vi "Show Cursors_Normal.vi"(6 "Cursor Options":T1={"font"={"Font Name"="Arial", "Size"=14, "Strikeout?"=FALSE, "Italic?"=FALSE, "Underline?"=FALSE, "Outline?"=FALSE, "Shadow?"=FALSE, "Bold?"=FALSE}, "size"=1, "Timestamp"=enum."at TOP", "Vertical Line?"=TRUE, "Horizontal Line?"=TRUE, "alignment(left, top)"={"horizontal"=enum."left", "vertical"=enum."center"}, "TextFormat"=" %3$s\\n %2$.2f", "time format (%H:%M:%S)"="%H:%M:%S"} {"size" min=1 max=50}, 7 "Index":i32, 8 "error in (no error)":errorcluster, 9 "Coords":T2, 10 "XY Graph":refnum<vi>, 11 "input picture":picture) -> (0 "error out":errorcluster, 3 "output picture":picture)   [LabVIEW 2018]
doc: "Shows real time cursors overlayed in a graph, using just one mouse move event case. The options for the cursors can be highly customized to set up a unique cursor style.\n\nUsage: Place this inside an event structure on any XY graph, in the \"Mouse Move\" event case. Set the options as an input cluster to override the defaults. The output picture control would typically be connected to the XY Graph's \"PlotImages.Front\" property item.\n\nCursor Options\n<b>Horizontal Line?</b> - Draws a horizontal line to intersect each plot\n<b>Verticle Line?</b> - Draws a verticle line at the mouse location to highlight the cursor location (typically on the time scale)\n<b>Timestamp</b> - Sets where to display the timestamp (if you want it at the top or bottom) Used best with the verticle line turned on.\n<b>Font</b> - Setup the font for displaying the cursor text\n<b>Alignment</b> - Sets the alignment options for the text relative to the cursor point\n<b>TextFormat</b> - Sets the text display format at the cursor points to show. Three input parameters are available for the text, which can be accessed using parameter numbers.\ninputs: \n1$ - Timestamp at cursor locations\n2$ - Value of the plot\n3$ - Name of the plot\n\nExamples: $2$.2f\\n\\n%1$s\nThis shows the value of the plot with 2 decimal places. A blank line, then the name of the plot"
uses:
  <vilib>/Utility/miscctls.llb/LVPoint32TypeDef.ctl
  CursorOptions.ctl
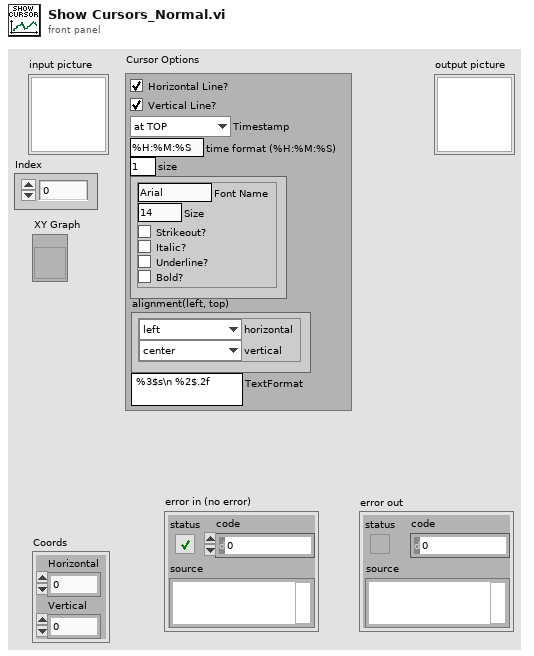
[diagram p1: front panel]
types:
  T1 = typedef "CursorOptions.ctl" = cluster{"font":cluster{"Font Name":string, "Size":i16, "Strikeout?":bool, "Italic?":bool, "Underline?":bool, "Outline?":bool, "Shadow?":bool, "Bold?":bool}, "size":i16, "Timestamp":enum16{"at TOP", "at BOTTOM", "none"}, "Vertical Line?":bool, "Horizontal Line?":bool, "alignment(left, top)":cluster{"horizontal":enum16{"left", "center", "right"}, "vertical":enum16{"top", "center", "bottom"}}, "TextFormat":string, "time format (%H:%M:%S)":string}
  T2 = typedef "LVPoint32TypeDef.ctl" = cluster{"Horizontal":i32, "Vertical":i32}
  T3 = enum16{"User-specified Font", "Application Font", "System Font", "Dialog Font"}
  T4 = cluster{"horizontal":enum16{"left", "center", "right"}, "vertical":enum16{"top", "center", "bottom"}}
  T5 = cluster{"Font Name":string, "Size":i16, "Strikeout?":bool, "Italic?":bool, "Underline?":bool, "Outline?":bool, "Shadow?":bool, "Bold?":bool}
  T6 = typedef "LVRectTypeDef.ctl" = cluster{"Left":i16, "Top":i16, "Right":i16, "Bottom":i16}
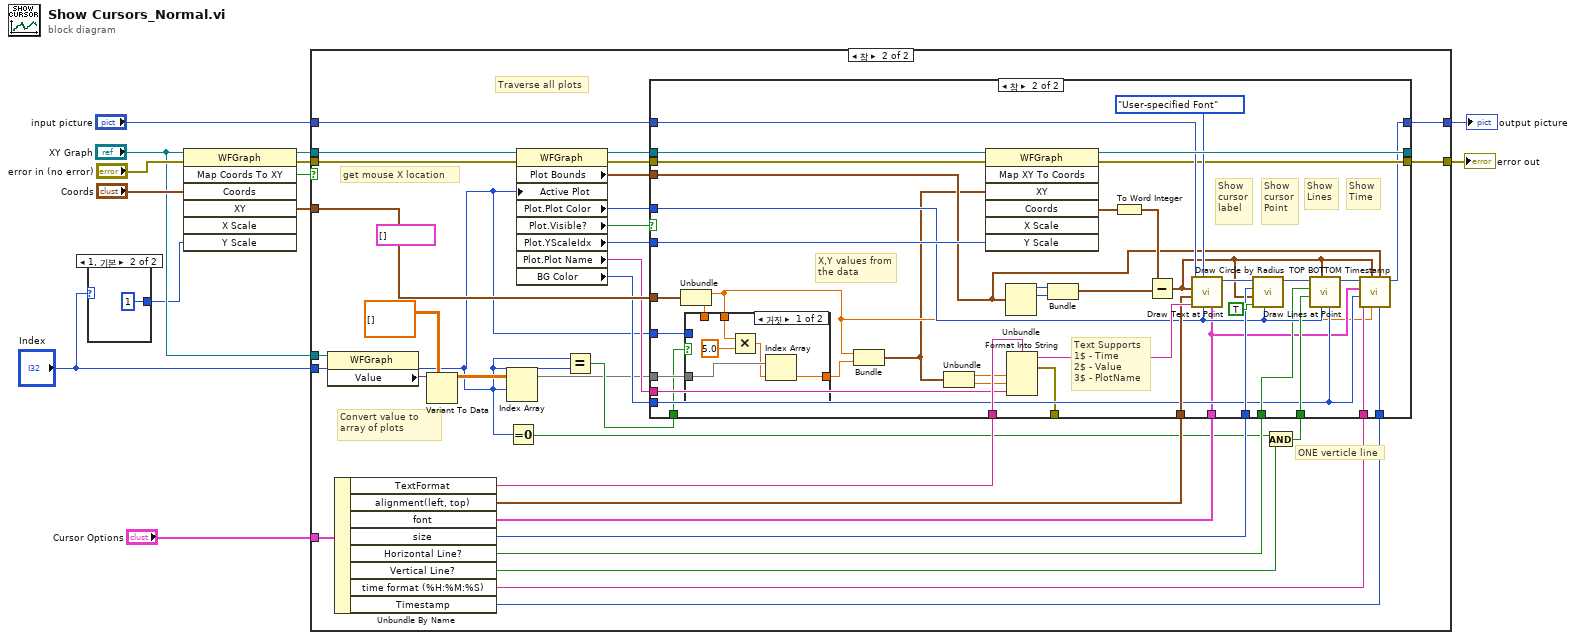
[diagram p0: block diagram]
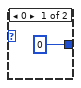
[diagram p2: hidden frame]
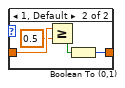
[diagram p6: hidden frame]
diagram:
  n1 = case shown="1, 기본" "Index" {
    tunnel: [0 1] -> w1
    frame 0 {
    }
    frame 1, Default {
    }
  }
  n2 = invoke on="Invoke Node" class="WFGraph" method="Map Coords To XY"(reference="XY Graph", error in="error in (no error)", "Coords"="Coords", "Y Scale"=w1) -> (reference out=w10:refnum<vi>, error out=w9:errorcluster, "Map Coords To XY"=w12:bool, "XY"=w13:cluster{"X":dbl, "Y":dbl})  [unwired: 3 in, 3 out]
  n3 = case shown="참" w12 {
    tunnel: w13 -> [_ w48]
    tunnel: w10 -> [_ w49]
    tunnel: [w16 w47] -> w5
    tunnel: w9 -> [w17 w46]
    tunnel: [w17 w45] -> w8
    tunnel: "input picture" -> [w16 w44]
    tunnel: "Cursor Options" -> [_ w36]
    tunnel: "XY Graph" -> [_ w34]
    tunnel: "Index" -> [_ w18]
    frame False {
      # "not in plot area.  clear the image"
    }
    frame True {
      (unwired) cluster{dbl[], dbl[]}[] []
      # "Traverse all plots"
      # "ONE verticle line"
      # "Convert value to array of plots"
      # "get mouse X location"
      n4 = property class="WFGraph"(reference=w34) -> ("Value"=w33:variant)  [unwired: 1 in, 2 out]
      n5 = Unbundle By Name(w36) -> ("TextFormat"=w43:string, "alignment(left, top)"=w42:T4, "font"=w41:T5, "size"=w40:i16, "Horizontal Line?"=w39:bool, "Vertical Line?"=w38:bool, "time format (%H:%M:%S)"=w32:string, "Timestamp"=w37:enum16{"at TOP", "at BOTTOM", "none"})
      n6 = Variant To Data(type=dbl[][] [], Variant=w33) -> (data=w35:dbl[][])  [unwired: 1 in, 1 out]
      n7 = Index Array(array=w35, index (row)=w18) -> (element=w19:dbl[])  [unwired: 1 in]
      n8 = Equal To 0?(x=w18) -> (x = 0?=w21:bool)
      n9 = property on="Property Node" class="WFGraph"(reference=w49, error in=w46, "Active Plot"=w18) -> (reference out=w29:refnum<vi>, error out=w26:errorcluster, "Plot Bounds"=w30:T6, "Plot.Plot Color"=w28:u32, "Plot.Visible?"=w27:bool, "Plot.YScaleIdx"=w25:u32, "Plot.Plot Name"=w23:string, "BG Color"=w22:u32)
      n10 = Equal?(x=w18, y=w18) -> (x = y?=w20:bool)
      n11 = And(x=w21, y=w38) -> (x .and. y?=w24:bool)
      n12 = case shown="참" w27 {
        tunnel: w30 -> [_ w65]
        tunnel: [w52 w89] -> _
        tunnel: w19 -> [_ w60]
        tunnel: w48 -> [_ w56]
        tunnel: w44 -> [w51 w88]
        tunnel: w29 -> [w52 w86]
        tunnel: [w51 w69] -> w47
        tunnel: w28 -> [_ w74]
        tunnel: w26 -> [w50 w82]
        tunnel: [w50 w81] -> w45
        tunnel: w25 -> [_ w80]
        tunnel: w40 -> [_ w79]
        tunnel: w42 -> [_ w78]
        tunnel: w41 -> [_ w63]
        tunnel: w43 -> [_ w77]
        tunnel: w39 -> [_ w73]
        tunnel: w24 -> [_ w76]
        tunnel: w23 -> [_ w70]
        tunnel: w37 -> [_ w67]
        tunnel: w22 -> [_ w64]
        tunnel: [_ w62] -> _
        tunnel: w32 -> [_ w61]
        tunnel: w20 -> [_ w55]
        tunnel: w18 -> [_ w53]
        frame False {
          # "plot is not visible, so don't show the cursor for it."
        }
        frame True {
          # "Show\nTime"
          # "Show\nLines"
          # "Show\ncursor\nPoint"
          # "Show\ncursor\nlabel"
          # "Text Supports\n1$ - Time\n2$ - Value\n3$ - PlotName"
          # "X,Y values from the data"
          n13 = Unbundle(w56) -> ("X"=w59:dbl, "Y"=w54:dbl)
          n14 = case shown="거짓" w55 {
            tunnel: w60 -> [w99 _]
            tunnel: w59 -> [w98 _]
            tunnel: [w95 w101] -> w58
            tunnel: w54 -> [_ w100]
            tunnel: w53 -> [_ w102]
            frame False {
              n15 = Multiply(x=w98, y=5.0) -> (x*y=w97:dbl)
              n16 = Index Array(array=w99, index=w97) -> (element=w95:dbl)
            }
            frame True {
              n17 = case shown="0" w102 {
                tunnel: [w103 w104] -> w101
                tunnel: w100 -> [w103 w107]
                frame 0 {
                }
                frame 1, Default {
                  n18 = Greater Or Equal?(x=w107, y=0.5) -> (x >= y?=w105:bool)
                  n19 = Boolean To (0,1)(Boolean=w105) -> (0, 1=w104:i16)
                }
              }
            }
          }
          n20 = Bundle("X"=w59, "Y"=w58) -> (w57:cluster{"X":dbl, "Y":dbl})  [unwired: 1 in]
          n21 = Unbundle(w57) -> ("X"=w72:dbl, "Y"=w71:dbl)
          n22 = invoke on="Invoke Node" class="WFGraph" method="Map XY To Coords"(reference=w86, error in=w82, "XY"=w57, "Y Scale"=w80) -> (reference out=w89:refnum<vi>, error out=w81:errorcluster, "Coords"=w94:T2)  [unwired: 3 in, 4 out]
          n23 = Unbundle(w65) -> ("Left"=w92:i16, "Top"=w93:i16)  [unwired: 2 out]
          n24 = Format Into String(format string=w77, w72, w71, w70) -> (resulting string=w87:string, error out=w62:errorcluster)  [unwired: 2 in]
          n25 = Bundle("Left"=w92, "Top"=w93) -> (w90:cluster{"Left":i16, "Top":i16})  [unwired: 1 in]
          n26 = To Word Integer(number=w94) -> (16bit integer=w91:cluster{"Horizontal":i16, "Vertical":i16})
          n27 = Subtract(x=w91, y=w90) -> (x-y=w66:cluster{i16, i16})
          n28 = call <vilib>:"Draw Text at Point.vi"("[user-specified font]"=w63, "text color(black)"=w74, "desired font(Application)"=T3."User-specified Font", "text"=w87, "alignment(left, top)"=w78, "origin"=w66, "picture"=w88) -> ("new picture"=w85:picture)  [unwired: 3 in, 1 out]
          n29 = call <vilib>:"Draw Circle by Radius.vi"("color(black)"=w74, "fill?(F)"=TRUE, "pixel center"=w66, "radius"=w79, "picture"=w85) -> ("new picture"=w75:picture)  [unwired: 6 in]
          n30 = call "Draw Lines at Point.vi"("GraphBGK"=w64, "color(black)"=w74, "pixel center"=w66, "Vertical Line?"=w76, "Horizontal Line?"=w73, "new picture in"=w75) -> ("new picture out"=w68:picture)  [unwired: 5 in]
          n31 = call "TOP BOTTOM Timestamp.vi"("Format"=w67, "Rect"=w65, "Timestamp"=w59, "pixel center"=w66, "time format (%H:%M:%S)"=w61, "GraphBGK"=w64, "font"=w63, "new picture in"=w68) -> ("new picture out"=w69:picture)  [unwired: 3 in]
        }
      }
    }
  }
  "error out" <- w8
  "output picture" <- w5
